vi "CameraGetData.vi"(8 "error in (no error)":errorcluster, 10 "keep open?":bool, 11 "NIvision in":refnum<class "IMAQdx.lvclass">) -> (0 "error out":errorcluster, 2 "image_data":u16[][][](array[numeric]), 3 "NIvision out":refnum<class "IMAQdx.lvclass">)   [LabVIEW 2010, in "IMAQdx.lvclass"]
uses:
  <userlib>/bias/classes/IMAQdx/IMAQdx.lvclass
  <userlib>/bias/classes/IMAQdx/IMAQdx.lvclass/IMAQdx.ctl
  <vilib>/vision/driver/IMAQdx.llb/IMAQdx Buffer Number Mode.ctl
  <vilib>/vision/driver/NI_Vision_Acquisition_Software.lvlib
  resource/objmgr/imaqdx.rc
  <userlib>/bias/c/imaging_tools.dll
panel:
  out "ValueDBL":dbl
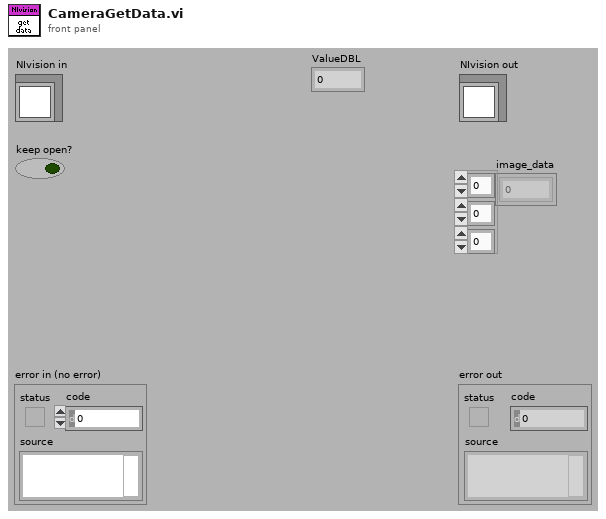
[diagram p1: front panel]
types:
  T1 = typedef "NI_Vision_Acquisition_Software.lvlib/IMAQdx Buffer Number Mode.ctl" = enum32{"Next", "Last", "Buffer Number"}
  T2 = typedef "IMAQdx.ctl" = refnum<k21>
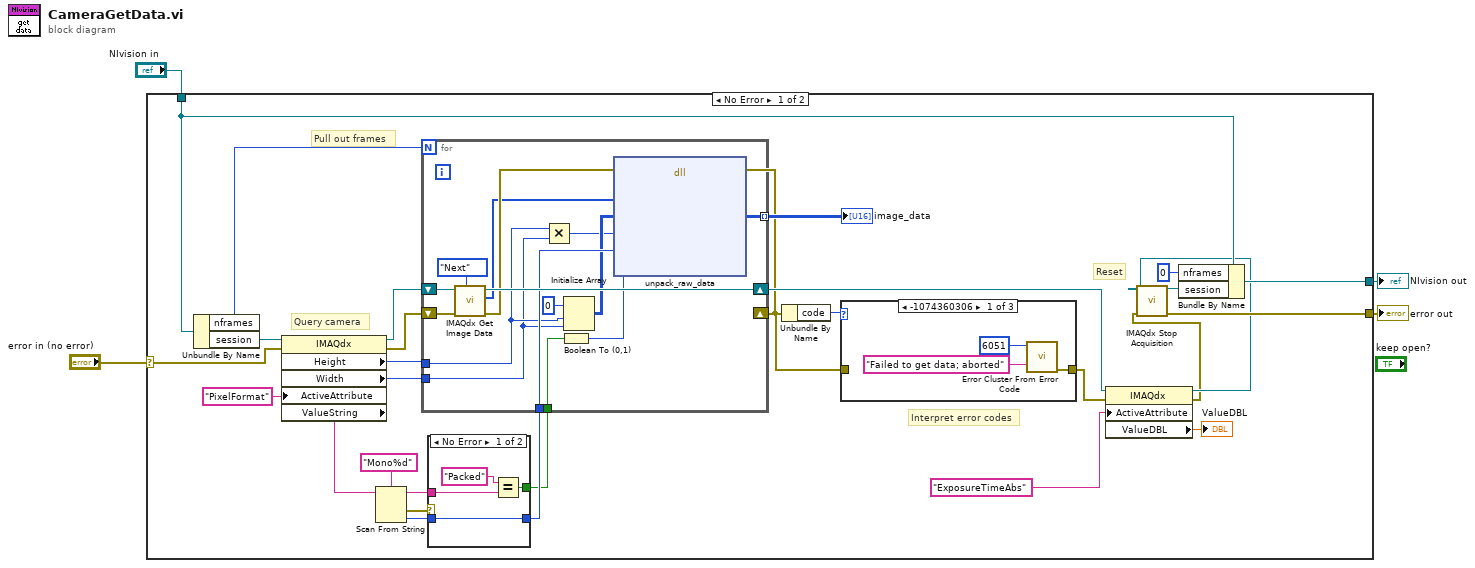
[diagram p0: block diagram]
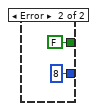
[diagram p2: hidden frame]
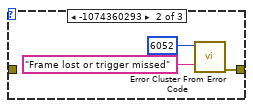
[diagram p3: hidden frame]
diagram:
  n1 = case shown="No Error" "error in (no error)" {
    selector: "error in (no error)" -> [w16 w63]
    tunnel: "NIvision in" -> [w30 w64]
    tunnel: [w15 w64] -> w2
    tunnel: [w13 w63] -> w1
    frame No Error {
      # "Query camera"
      # "Interpret error codes"
      # "Reset"
      # "Pull out frames"
      n2 = Unbundle By Name(w30) -> ("nframes"=w29:i32, "session"=w12:refnum<k21>)
      n3 = property class="IMAQdx"(reference=w12, error in=w16, "ActiveAttribute"="PixelFormat") -> (reference out=w11:refnum<k21>, error out=w33:errorcluster, "Height"=w32:u32, "Width"=w31:u32, "ValueString"=w23:string)
      n4 = Scan From String(format string="Mono%d", input string=w23) -> (remaining string=w22:string, error out=w21:errorcluster, output 1=w20:i32)  [unwired: 3 in, 1 out]
      n5 = case shown="No Error" w21 {
        tunnel: w22 -> [w37 _]
        tunnel: [w35 FALSE] -> w18
        tunnel: [w34 8] -> w19
        tunnel: w20 -> [w34 _]
        frame No Error {
          n6 = Equal?(x="Packed" ("format string"), y=w37) -> (x = y?=w35:bool)
        }
        frame Error {
        }
      }
      n7 = for {
        N: w29 -> [_]
        tunnel: [w57] -> w17 mode=indexing
        shift-right: [w61] -> w10
        shift-left: w11 -> [w62]
        shift-right: [w56] -> w26
        shift-left: w33 -> [w60]
        tunnel: w32 -> [w55]
        tunnel: w31 -> [w54]
        tunnel: w19 -> [w59]
        tunnel: w18 -> [w58]
        n8 = call <vilib>:"IMAQdx Get Image Data.vi"("Buffer Number Mode (Next)"=IMAQdx_Buffer_Number_Mode."Next", "error in"=w60, "Session In"=w62) -> ("error out"=w48:errorcluster, "Image Data Array"=w47:u8[], "Session Out"=w61:T2)  [unwired: 5 in, 1 out]
        n9 = Multiply(x=w55, y=w54) -> (x*y=w50:u32)
        n10 = Boolean To (0,1)(Boolean=w58) -> (0, 1=w49:i16)
        n11 = Initialize Array(u16 0 ("element"), w55, w54) -> (w51:u16[][])
        n12 = dll-call lib="C:/Program Files (x86)/National Instruments/LabVIEW 2010/user.lib/bias/c/imaging_tools.dll" fn="unpack_raw_data"(error in=w48, "in"=w47, "out"=w51, "N"=w50, "bits"=w59, "packed"=w49) -> (error out=w56:errorcluster, "out"=w57:u16[][])  [unwired: 7 in, 1 out]
      }
      "image_data" <- w17
      n13 = Unbundle By Name(w26) -> ("code"=w27:i32)
      n14 = case shown="-1074360306" w27 {
        tunnel: [w40 w43 w46] -> w8
        tunnel: w26 -> [_ _ w46]
        frame -1074360306 {
          n15 = call <vilib>:"Error Cluster From Error Code.vi"("error message (\"\")"="Failed to get data; aborted" ("error message (\"\")"), "error code (0)"=6051) -> ("error out"=w40:errorcluster)  [unwired: 7 in]
        }
        frame -1074360293 {
          n16 = call <vilib>:"Error Cluster From Error Code.vi"("error message (\"\")"="Frame lost or trigger missed" ("error message (\"\")"), "error code (0)"=6052) -> ("error out"=w43:errorcluster)  [unwired: 7 in]
        }
        frame Default {
        }
      }
      n17 = property class="IMAQdx"(reference=w10, error in=w8, "ActiveAttribute"="ExposureTimeAbs") -> (reference out=w9:refnum<k21>, error out=w7:errorcluster, "ValueDBL"=→"ValueDBL":dbl)
      n18 = call <vilib>:"IMAQdx Stop Acquisition.vi"("error in"=w7, "Session In"=w9) -> ("error out"=w13:errorcluster, "Session Out"=w14:T2)  [unwired: 8 in]
      n19 = Bundle By Name(cluster=w30, "nframes"=0, "session"=w14) -> (w15:refnum<class "IMAQdx.lvclass">)
    }
    frame Error {
    }
  }
  "NIvision out" <- w2
  "error out" <- w1
